vi "Anritsu VNA Read Number of Available Channels.vi"(7 "Anritsu VNA":T1, 8 "error in (no error)":errorcluster, 11 "VISA Resource Name":refnum<visa-resource-name>) -> (0 "error out":errorcluster, 2 "Number of Channels":i8, 3 "dup VISA Resource Name":refnum<visa-resource-name>)   [LabVIEW 2011]
doc: "This VI for the HP 8753 is used to read the sweep type.\n\n0 LINEAR FREQ\n1 LOG FREQ\n2 LIST FREQ\n3 CW TIME\n4 POWER SWEEP"
uses:
  TypeDefs/Anritsu VNA Instrument Info.ctl
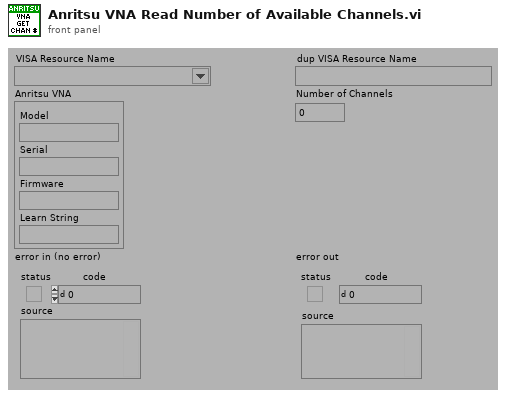
[diagram p1: front panel]
types:
  T1 = typedef "Anritsu VNA Instrument Info.ctl" = cluster{"Model":string, "Serial":string, "Firmware":string, "Learn String":string}
  T2 = typedef "Anritsu VNA Model.ctl" = enum16{"Not Supported", "37XXXX", "MS20XXX", "MS462XX", "MS464XX"}
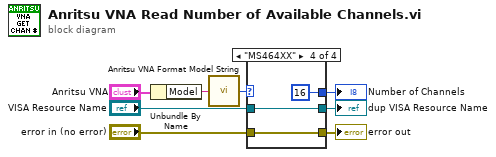
[diagram p0: block diagram]
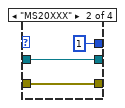
[diagram p3: hidden frame]
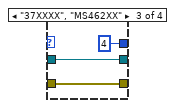
[diagram p4: hidden frame]
diagram:
  n1 = Unbundle By Name("Anritsu VNA") -> ("Model"=w2:string)
  n2 = call "Anritsu VNA Format Model String.vi"("Model"=w2) -> ("Model"=w1:T2)
  n3 = case shown="\"MS464XX\"" w1 {
    tunnel: "VISA Resource Name" -> [w10 w12 w15 w18]
    tunnel: "error in (no error)" -> [w9 w13 w16 w19]
    tunnel: [w9 w13 w16 w19] -> w7
    tunnel: [_ i8 1 i8 4 i8 16] -> w6
    tunnel: [w10 w12 w15 w18] -> w4
    frame "Not Supported" {
    }
    frame "MS20XXX" {
    }
    frame "37XXXX", "MS462XX" {
    }
    frame "MS464XX" {
    }
  }
  "Number of Channels" <- w6
  "dup VISA Resource Name" <- w4
  "error out" <- w7
